vi "init.vi"(8 "error in (no error)":errorcluster, 11 "StepperMotorTC in":refnum<class "StepperMotorTC.lvclass">) -> (0 "error out":errorcluster, 3 "StepperMotorTC out":refnum<class "StepperMotorTC.lvclass">)   [LabVIEW 2013, in "StepperMotorTC.lvclass"]
uses:
  StepperMotorTC.lvclass
  <userlib>/Common/Devices/StepperMotor/Config/StepperMotor.ctl
  <userlib>/Common/Devices/StepperMotor/StepperMotor/StepperMotor.lvclass/StepperMotor.ctl
  <userlib>/Common/Devices/StepperMotor/StepperMotor/StepperMotor.lvclass
  <userlib>/Common/Devices/StepperMotor/StepperMotor.lvlib
  ConfigurationThisComponent/ConfigurationThisComponent.lvclass
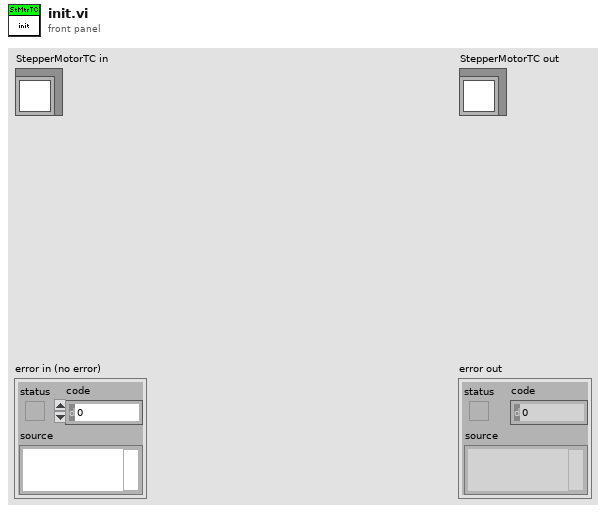
[diagram p1: front panel]
types:
  T1 = typedef "StepperMotor.lvlib/StepperMotor.ctl" = cluster{"Maximum Step Rate":dbl[unit]}
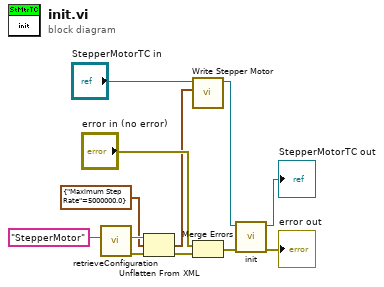
[diagram p0: block diagram]
diagram:
  n1 = call "retrieveConfiguration.vi"("configName"="StepperMotor") -> ("error out"=w9:errorcluster, "xmlConfig"=w8:string)  [unwired: 8 in, 1 out]
  n2 = Unflatten From XML(xml string=w8, type=T1 {"Maximum Step Rate"=5000000.0} ("Stepper Motor"), error in (no error)=w9) -> (value=w1:T1, error out=w5:errorcluster)
  n3 = call <userlib>:"Write Stepper Motor.vi"("Stepper Motor"=w1, "StepperMotor in"="StepperMotorTC in") -> ("StepperMotor out"=w2:refnum<class "StepperMotorTC.lvclass">)  [unwired: 9 in]
  n4 = Merge Errors("error in (no error)", w5) -> (w4:errorcluster)
  n5 = call-parent "init.vi"("error in (no error)"=w4, "StepperMotor in"=w2) -> ("error out"=→"error out":errorcluster, "StepperMotor out"=→"StepperMotorTC out":refnum<class "StepperMotorTC.lvclass">)  [unwired: 8 in]
